vi "SCC-TC0x Calculate Temperatures.vi"(5 "TC0x Gain":dbl=100.0 format="%.2f", 6 "Output Temperature Unit":u16(ring) items=["Celsius", "Fahrenheit", "Kelvin", "Rankine"], 7 "ThermocoupleType":u16(ring)=2 items=["B", "E", "J", "K", "R", "S", "T", "N"], 10 "CJC Voltage":dbl format="%.4f", 11 "T/C Voltage":dbl format="%.4f") -> (1 "Open T/C":bool, 2 "CJ Temperature":dbl=25.0 format="%0.2f", 3 "T/C Temperature":dbl=25.0 format="%0.2f")   [LabVIEW 2013]
doc: "DESCRIPTION:\nThis vi was cloned from the SCC-TC0x.vi which read the A/D and converted to temperature units. This vi simply takes the thermocouple and cold junction voltages in, and outputs the their temperatures in the appropriate units. An open T/C Boolean is also available. AutoCon, 7/05"
panel:
  # "This vi was cloned from the NI SCC-TC0x.vi - removed DAQ calls and\nmade it a simple T/C converter - AutoCon, 7/2005"
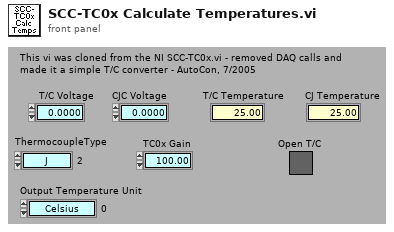
[diagram p1: front panel]
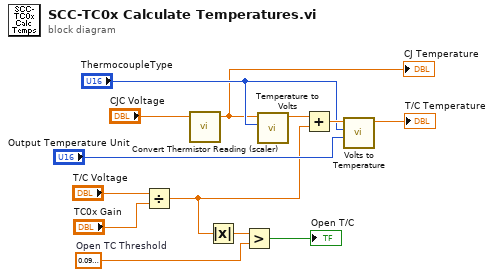
[diagram p0: block diagram]
diagram:
  w9 = sgl 0.09  # Open TC Threshold
  n1 = Divide(x="T/C Voltage", y="TC0x Gain") -> (x/y=w7:dbl)
  n2 = call "Convert Thermistor Reading (scaler).vi"("Voltage"="CJC Voltage") -> ("Temperature"=w1:sgl)  [unwired: 6 in]
  "CJ Temperature" <- w1
  n3 = Absolute Value(x=w7) -> (abs(x)=w8:dbl)
  n4 = Greater?(x=w8, y=w9) -> (0:→"Open T/C":bool)
  n5 = call "Temperature to Volts.vi"("ThermocoupleType"="ThermocoupleType", "Temperature"=w1) -> ("Thermocouple Voltage"=w13:sgl)  [unwired: 5 in]
  n6 = Add(x=w13, y=w7) -> (x+y=w12:dbl)
  n7 = call "Volts to Temperature.vi"("Temperature Units"="Output Temperature Unit", "ThermocoupleType"="ThermocoupleType", "Thermocouple Voltage"=w12) -> ("Temperature"=→"T/C Temperature":sgl)  [unwired: 4 in]
